vi "get_speed.vi"(8 "error in (no error)":errorcluster caption="错误输入（无错误）", 11 "StepMotor 输入":refnum<class "StepMotor.lvclass">) -> (0 "error out":errorcluster caption="错误输出", 2 "speed":i32, 3 "StepMotor 输出":refnum<class "StepMotor.lvclass">)   [LabVIEW 2016, in "MotionControl.lvlib" / "StepMotor.lvclass"]
uses:
  <userlib>/MotionControl/StepMotor/StepMotor.lvclass
  <userlib>/MotionControl/StepMotor/StepMotor.lvclass/StepMotor.ctl
  <userlib>/UISimCanFunc_wrapper/UISimCanFunc_wrapper.lvlib
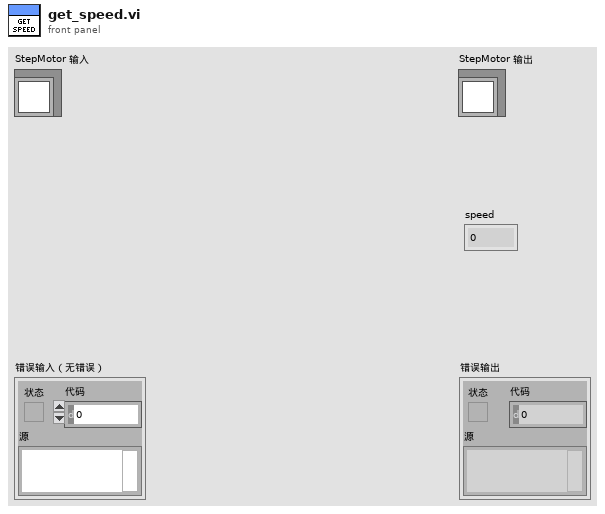
[diagram p1: front panel]
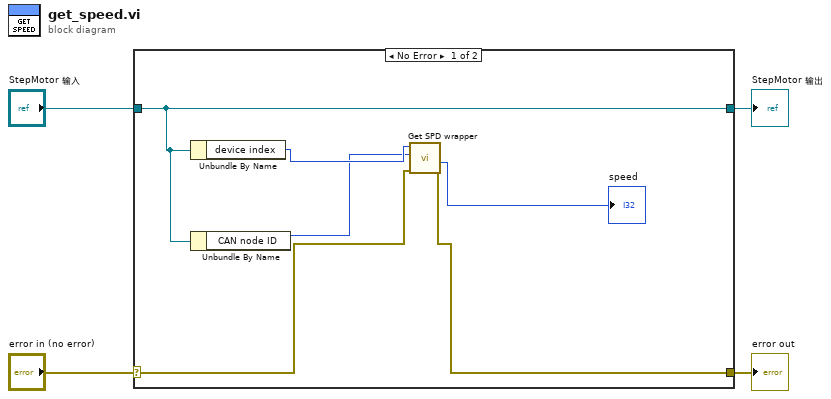
[diagram p0: block diagram]
diagram:
  n1 = case shown="No Error" "error in (no error)" {
    selector: "error in (no error)" -> [w6 w12]
    tunnel: [w5 w12] -> w3
    tunnel: [w10 w11] -> w1
    tunnel: "StepMotor 输入" -> [w10 w11]
    frame No Error {
      n2 = Unbundle By Name(w10) -> ("device index"=w9:u32)
      n3 = Unbundle By Name(w10) -> ("CAN node ID"=w8:u32)
      n4 = call <userlib>:"Get SPD wrapper.vi"("error in (no error)"=w6, "dwCanNodeId"=w8, "dwDevIndex"=w9) -> ("error out"=w5:errorcluster, "pRtnValue out"=→"speed":i32)  [unwired: 6 in, 1 out]
    }
    frame Error {
    }
  }
  "error out" <- w3
  "StepMotor 输出" <- w1
